vi "AcquireWaveformsFpgaWithTach.vi"(8 "error in (no error)":errorcluster, 11 "923x Acquisition Config":T1={"Acq"=FALSE, "NumberOfModules"=0, "Dynamic FPGA VI Ref"=refnum, "KeyphasorX3"=[], "FixedSizeX32"={"EnabledChannels"=[], "Sensitivity"=[], "InputConfig"=[]}, "SamplingInfo"={"Number of Channels"=4, "Sampling Rate"=4.0, "Channels"=[], "Units"=[], "Offsets"=[]}, "Normal Mode Sample Rate"=0.0, "BlockSize (sec)"=0.0, "Samples To Read (per chan)"=0, "RunningAcquisitionLength"=0.0, "Settling Time"=0.0, "Waveform Groups"=[], "Acquisition Block Number"=0, "Device Name"="", "ValidConfig"=FALSE, "Last Dynamic Module"="", "HighPassFilterState"=[], "Low Frequency Cutoff"=[], "BurstMode"={"Acquisition Time"=0.0, "Sample Rate"=0.0}} {"HighPassFilterState"."Filter State" format="%.2f"; "HighPassFilterState"."IIR Filter Cluster"."Forward Coefficients" format="%.2f"; "HighPassFilterState"."IIR Filter Cluster"."Reverse Coefficients" format="%.2f"; "FixedSizeX32"."InputConfig" items=["AC Coupled", "DC Coupled", "IEPE AC Coupled"]}) -> (0 "error out":errorcluster, 1 "OSClkStart":dbl, 2 "Pulse Positions Array":T10[](array[typedef]), 3 "Waveforms":waveform(sgl)[](array[waveform]))   [LabVIEW 2017, in "CmsAcquisition.lvlib"]
uses:
  <vilib>/addons/InsightCM/Devices/Shared/Cms/CmsAcquisition/CmsAcquisition.lvlib
  <vilib>/addons/InsightCM/Utilities/Analysis/Shared/controls/PulsePositions.ctl
  <vilib>/addons/InsightCM/Devices/Shared/Cms/CmsAcquisition/controls/Configuration.ctl
  <vilib>/addons/InsightCM/Devices/Shared/Cms/CmsAcquisition/controls/TachometerConfig.ctl
  <vilib>/addons/InsightCM/Devices/Shared/Cms/CmsAcquisition/controls/FixedSizeArrays.ctl
  <vilib>/LabVIEW Targets/FPGA/cRIO/shared/nicrio_ModuleControls/nicrio_cRIO-9232_ConfigModeRing.ctl
  <vilib>/addons/InsightCM/Devices/Shared/Cms/cRIOWfmAcq/subVIs/RIO Wfm Cust Ctrls/rwfm_SamplingInfo.ctl
  <vilib>/addons/InsightCM/Devices/Shared/Cms/CmsAcquisition/controls/Group.ctl
  <vilib>/addons/InsightCM/Devices/Shared/Cms/CmsAcquisition/controls/Channel.ctl
  <vilib>/addons/InsightCM/Utilities/Analysis/Vibration/controls/HighPassFilterState.ctl
  <vilib>/addons/InsightCM/Devices/Shared/Cms/CmsAcquisition/controls/BurstMode.ctl
  <vilib>/addons/InsightCM/Devices/Shared/Cms/cRIOWfmAcq/cRIOWfmLib.lvlib
  <vilib>/addons/InsightCM/Utilities/Analysis/Shared/AnalysisHelper.lvlib
  <vilib>/addons/InsightCM/Utilities/Analysis/Vibration/VibrationAnalysisFunctions.lvlib
panel:
  in  "burst mode":bool
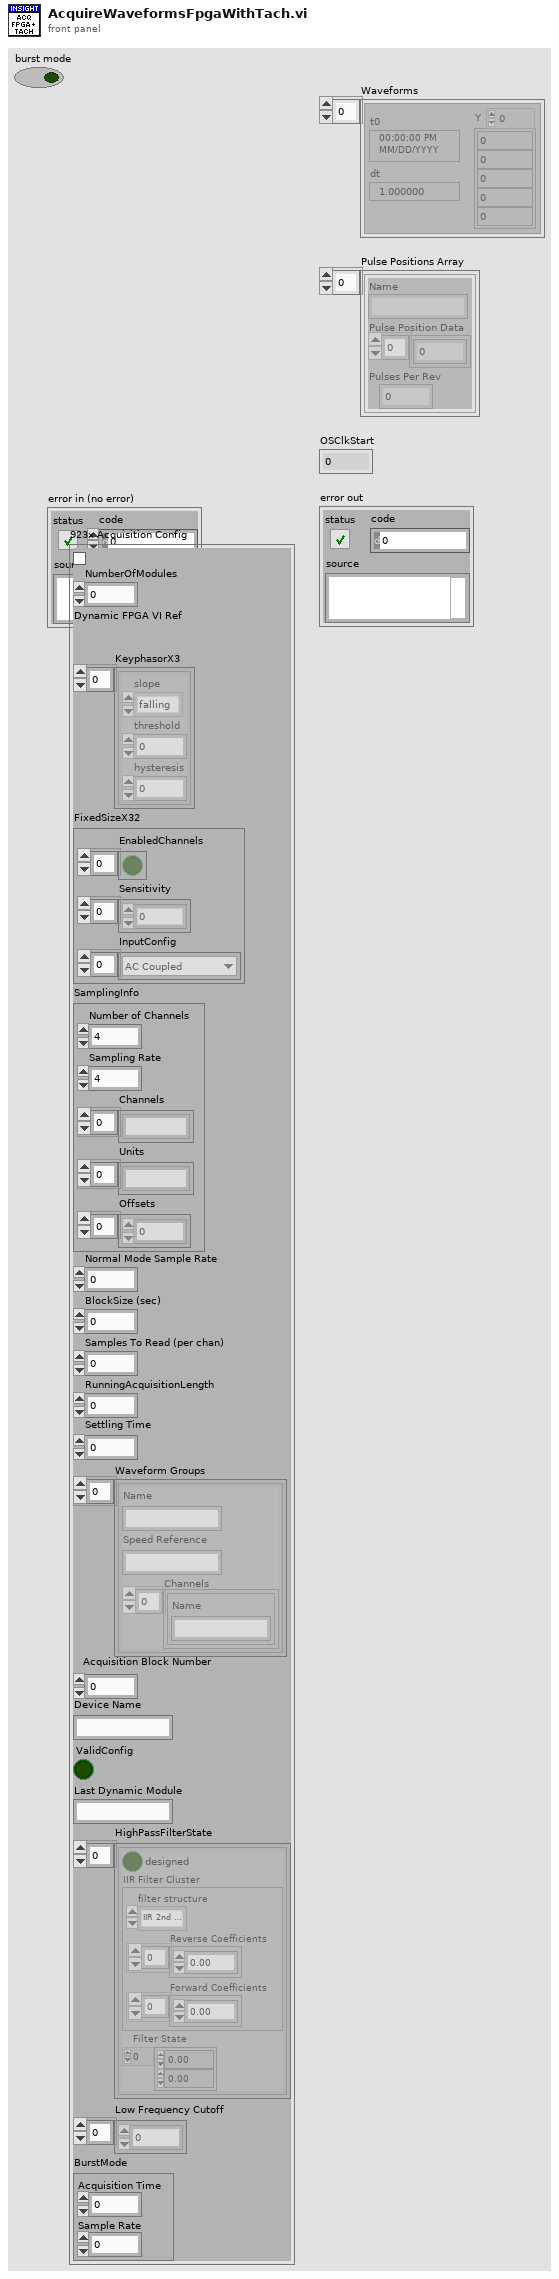
[diagram p1: front panel]
types:
  T1 = typedef "CmsAcquisition.lvlib/Configuration.ctl" = cluster{"Acq":bool, "NumberOfModules":i16, "Dynamic FPGA VI Ref":refnum<k20>, "KeyphasorX3":T2[], "FixedSizeX32":T3, "SamplingInfo":T5, "Normal Mode Sample Rate":dbl, "BlockSize (sec)":dbl, "Samples To Read (per chan)":i32, "RunningAcquisitionLength":dbl, "Settling Time":dbl, "Waveform Groups":T6[], "Acquisition Block Number":i32, "Device Name":string, "ValidConfig":bool, "Last Dynamic Module":string, "HighPassFilterState":T8[], "Low Frequency Cutoff":dbl[], "BurstMode":T9}
  T2 = typedef "CmsAcquisition.lvlib/TachometerConfig.ctl" = cluster{"slope":enum16{"falling", "rising"}, "threshold":dbl, "hysteresis":dbl}
  T3 = typedef "CmsAcquisition.lvlib/FixedSizeArrays.ctl" = cluster{"EnabledChannels":bool[], "Sensitivity":dbl[], "InputConfig":T4[]}
  T4 = typedef "nicrio_cRIO-9232_ConfigModeRing.ctl" = u8
  T5 = typedef "cRIOWfmLib.lvlib/rwfm_SamplingInfo.ctl" = cluster{"Number of Channels":i32, "Sampling Rate":dbl, "Channels":string[], "Units":string[], "Offsets":sgl[]}
  T6 = typedef "CmsAcquisition.lvlib/Group.ctl" = cluster{"Name":string, "Speed Reference":string, "Channels":T7[]}
  T7 = typedef "CmsAcquisition.lvlib/Channel.ctl" = cluster{"Name":string}
  T8 = typedef "VibrationAnalysisFunctions.lvlib/HighPassFilterState.ctl" = cluster{"designed":bool, "IIR Filter Cluster":cluster{"filter structure":enum32{"IIR 2nd Order", "IIR 4th Order"}, "Reverse Coefficients":dbl[], "Forward Coefficients":dbl[]}, "Filter State":dbl[]}
  T9 = typedef "CmsAcquisition.lvlib/BurstMode.ctl" = cluster{"Acquisition Time":dbl, "Sample Rate":dbl}
  T10 = typedef "AnalysisHelper.lvlib/PulsePositions.ctl" = cluster{"Name":string, "Pulse Position Data":dbl[], "Pulses Per Rev":i32}
  T11 = typedef "cRIOWfmLib.lvlib/rwfm_FPGARefTach.ctl" = refnum<k20>
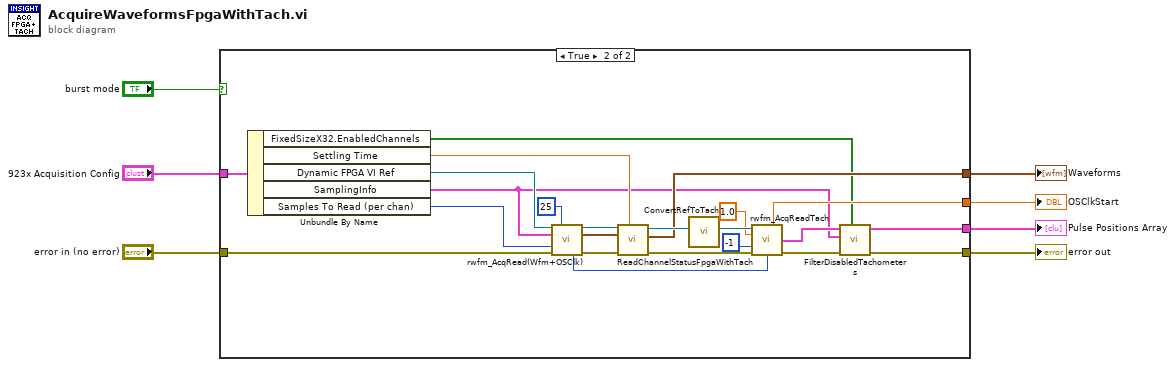
[diagram p0: block diagram]
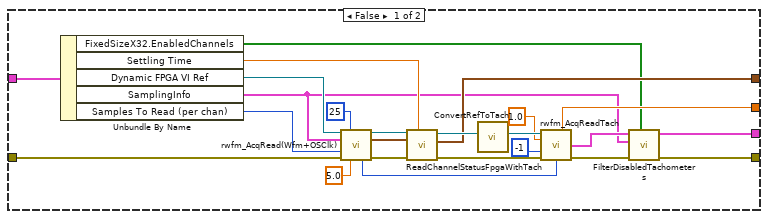
[diagram p2: hidden frame]
diagram:
  n1 = case shown="True" "burst mode" {
    tunnel: [w31 w54] -> w7
    tunnel: [w30 w53] -> w6
    tunnel: [w28 w51] -> w5
    tunnel: "error in (no error)" -> [w24 w47]
    tunnel: [w21 w44] -> w3
    tunnel: "923x Acquisition Config" -> [w16 w40]
    frame False {
      n2 = Unbundle By Name(w16) -> ("FixedSizeX32.EnabledChannels"=w14:bool[], "Settling Time"=w15:dbl, "Dynamic FPGA VI Ref"=w13:refnum<k20>, "SamplingInfo"=w11:T5, "Samples To Read (per chan)"=w12:i32)
      n3 = call <vilib>:"rwfm_AcqRead(Wfm+OSClk).vi"("Dynamic FPGA VI Reference"=w13, "Poll Time (ms)"=u32 25, "Sampling Info"=w11, "Samps Read per Chan"=w12, "error in"=w24, "Timeout (s)"=5.0) -> ("Dynamic FPGA VI Reference"=w20:refnum<k20>, "Wfm Data"=w25:waveform(sgl)[], "OSClkStart_U32"=w23:u32, "error out"=w9:errorcluster)  [unwired: 2 in, 4 out]
      n4 = call <vilib>:"ReadChannelStatusFpgaWithTach.vi"("IEPE settling blocks"=w15, "error in"=w9, "wfm data"=w25, "dynamic FPGA VI reference"=w20) -> ("error out"=w10:errorcluster, "wfm data"=w21:waveform(sgl)[], "dynamic FPGA VI reference"=w22:refnum<k20>)  [unwired: 5 in]
      n5 = call <vilib>:"ConvertRefToTach.vi"("FPGA Ref"=w22) -> ("FPGA Ref"=w17:T11)  [unwired: 10 in]
      n6 = call <vilib>:"rwfm_AcqReadTach.vi"("FPGA VI Reference"=w17, "acq block size (s)"=1.0, "Samps Read per Chan"=-1, "error in"=w10, "OSClkStart"=w23) -> ("OSClkStart"=w31:dbl, "Tachometer Pulses"=w29:T10[], "error out"=w27:errorcluster)  [unwired: 5 in, 3 out]
      n7 = call <vilib>:"FilterDisabledTachometers.vi"("channels enabled"=w14, "error in (no error)"=w27, "Sampling Info"=w11, "Pulse Positions Array in"=w29) -> ("error out"=w28:errorcluster, "Pulse Positions Array out"=w30:T10[])  [unwired: 6 in]
    }
    frame True {
      n8 = Unbundle By Name(w40) -> ("FixedSizeX32.EnabledChannels"=w38:bool[], "Settling Time"=w39:dbl, "Dynamic FPGA VI Ref"=w37:refnum<k20>, "SamplingInfo"=w35:T5, "Samples To Read (per chan)"=w36:i32)
      n9 = call <vilib>:"rwfm_AcqRead(Wfm+OSClk).vi"("Dynamic FPGA VI Reference"=w37, "Poll Time (ms)"=u32 25, "Sampling Info"=w35, "Samps Read per Chan"=w36, "error in"=w47) -> ("Dynamic FPGA VI Reference"=w43:refnum<k20>, "Wfm Data"=w48:waveform(sgl)[], "OSClkStart_U32"=w46:u32, "error out"=w33:errorcluster)  [unwired: 3 in, 4 out]
      n10 = call <vilib>:"ReadChannelStatusFpgaWithTach.vi"("IEPE settling blocks"=w39, "error in"=w33, "wfm data"=w48, "dynamic FPGA VI reference"=w43) -> ("error out"=w34:errorcluster, "wfm data"=w44:waveform(sgl)[], "dynamic FPGA VI reference"=w45:refnum<k20>)  [unwired: 5 in]
      n11 = call <vilib>:"ConvertRefToTach.vi"("FPGA Ref"=w45) -> ("FPGA Ref"=w41:T11)  [unwired: 10 in]
      n12 = call <vilib>:"rwfm_AcqReadTach.vi"("FPGA VI Reference"=w41, "acq block size (s)"=1.0, "Samps Read per Chan"=-1, "error in"=w34, "OSClkStart"=w46) -> ("OSClkStart"=w54:dbl, "Tachometer Pulses"=w52:T10[], "error out"=w50:errorcluster)  [unwired: 5 in, 3 out]
      n13 = call <vilib>:"FilterDisabledTachometers.vi"("channels enabled"=w38, "error in (no error)"=w50, "Sampling Info"=w35, "Pulse Positions Array in"=w52) -> ("error out"=w51:errorcluster, "Pulse Positions Array out"=w53:T10[])  [unwired: 6 in]
    }
  }
  "OSClkStart" <- w7
  "Pulse Positions Array" <- w6
  "error out" <- w5
  "Waveforms" <- w3
